vi "Configure Input Type.vi"   [LabVIEW 2017, in "Sefram DAS220.lvlib"]
doc: "Defines the selected input type according to your sensors : voltage, current, thermocouple, Pt100/1000, resistance.\nFor specials digitals channels from K1 to K4, you can select Frequency, Counter or PWM (duty cycle) measurement."
uses:
  <instrlib>/Sefram DAS220/Sefram DAS220.lvlib
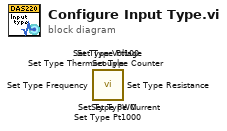
[diagram p0: block diagram]
diagram:
  n1 = call <instrlib>:"Set Type PWM.vi"() -> ()  [unwired: 10 in, 2 out]
  n2 = call <instrlib>:"Set Type Counter.vi"() -> ()  [unwired: 10 in, 2 out]
  n3 = call <instrlib>:"Set Type Frequency.vi"() -> ()  [unwired: 10 in, 2 out]
  n4 = call <instrlib>:"Set Type Resistance.vi"() -> ()  [unwired: 10 in, 2 out]
  n5 = call <instrlib>:"Set Type Pt1000.vi"() -> ()  [unwired: 10 in, 2 out]
  n6 = call <instrlib>:"Set Type Pt100.vi"() -> ()  [unwired: 10 in, 2 out]
  n7 = call <instrlib>:"Set Type Thermocouple.vi"() -> ()  [unwired: 10 in, 2 out]
  n8 = call <instrlib>:"Set Type Current.vi"() -> ()  [unwired: 10 in, 2 out]
  n9 = call <instrlib>:"Set Type Voltage.vi"() -> ()  [unwired: 10 in, 2 out]
